vi "tut1_main.vi"() -> ()   [LabVIEW 2014]
uses:
  <vilib>/measure/NI_MABase.lvlib
panel:
  in  "L":dbl(slide)=2e-06 min=1e-06 max=0.001 step=1e-07 scale=1e-06..0.001 scale format="%#.6p"
  out "Current Graph":waveform(dbl)[](graph)
  out "Voltage Graph":waveform(dbl)[](graph)
  out "Control Signal":waveform(dbl)[](graph)
  in  "DutyCycle":dbl(slide)=50.0 caption="Duty Cycle (%)" min=0.0 max=100.0 step=1.0 scale=0.0..100.0 scale format="%#.6p"
  in  "Frequency":dbl(slide)=50.0 caption="Signal Frequency (Hz)" min=0.0 max=5000.0 step=1.0 scale=0.0..100.0 scale format="%#.6p"
  in  "V":dbl(slide)=10.0 caption="Signal Voltage (V)" min=0.0 max=20.0 step=0.1 scale=0.0..20.0 scale format="%#.6p"
  in  "C":dbl(slide)=2e-06 min=1e-06 max=0.001 step=1e-07 scale=1e-06..0.001 scale format="%#.6p"
  in  "R":dbl(slide)=500.0 min=10.0 max=100000.0 step=1.0 scale=10.0..100000.0 scale format="%#.6p"
  in  "stop":bool
  # "PSI3214"
  # "Laboratório de \nInstrumentação Elétrica"
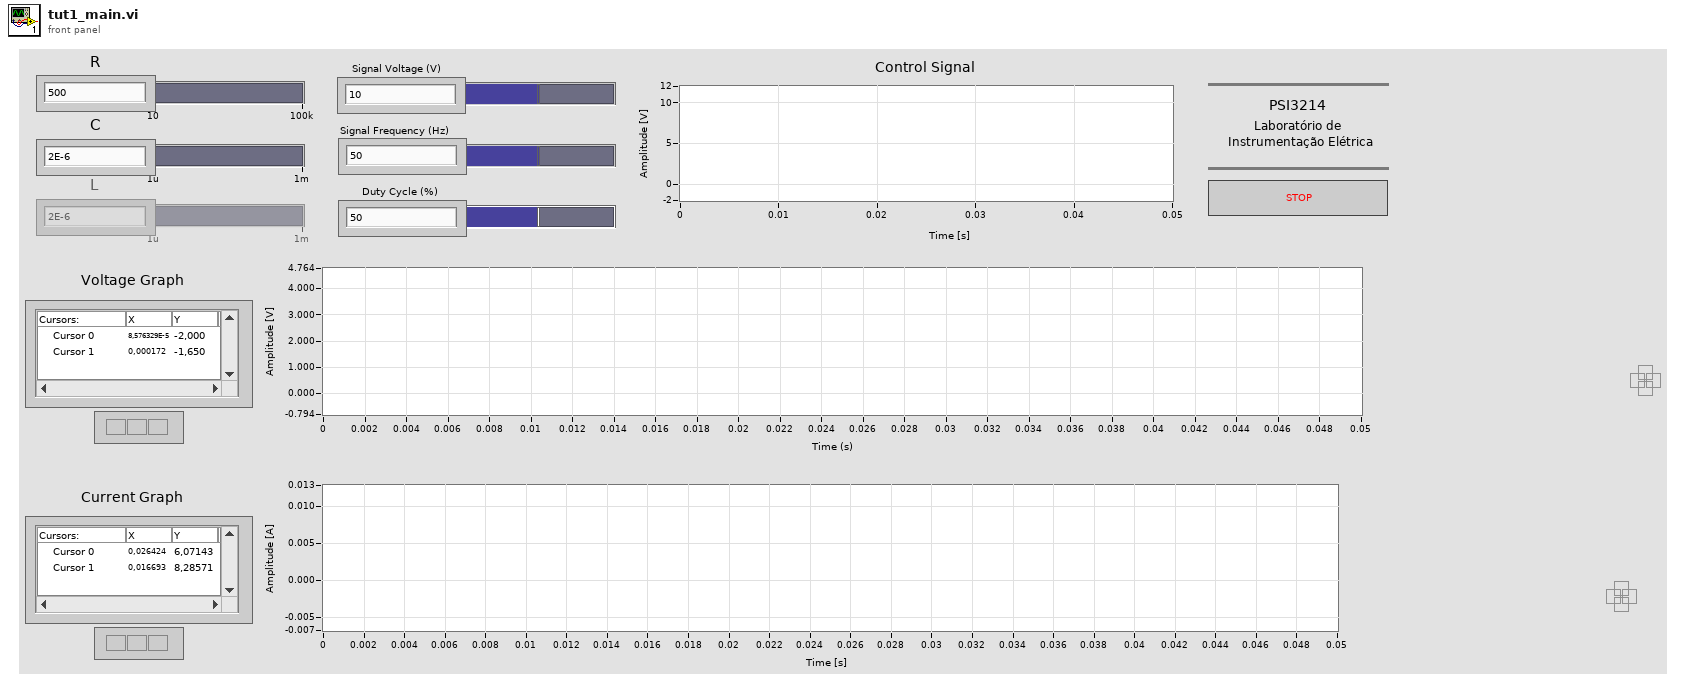
[diagram p1: front panel]
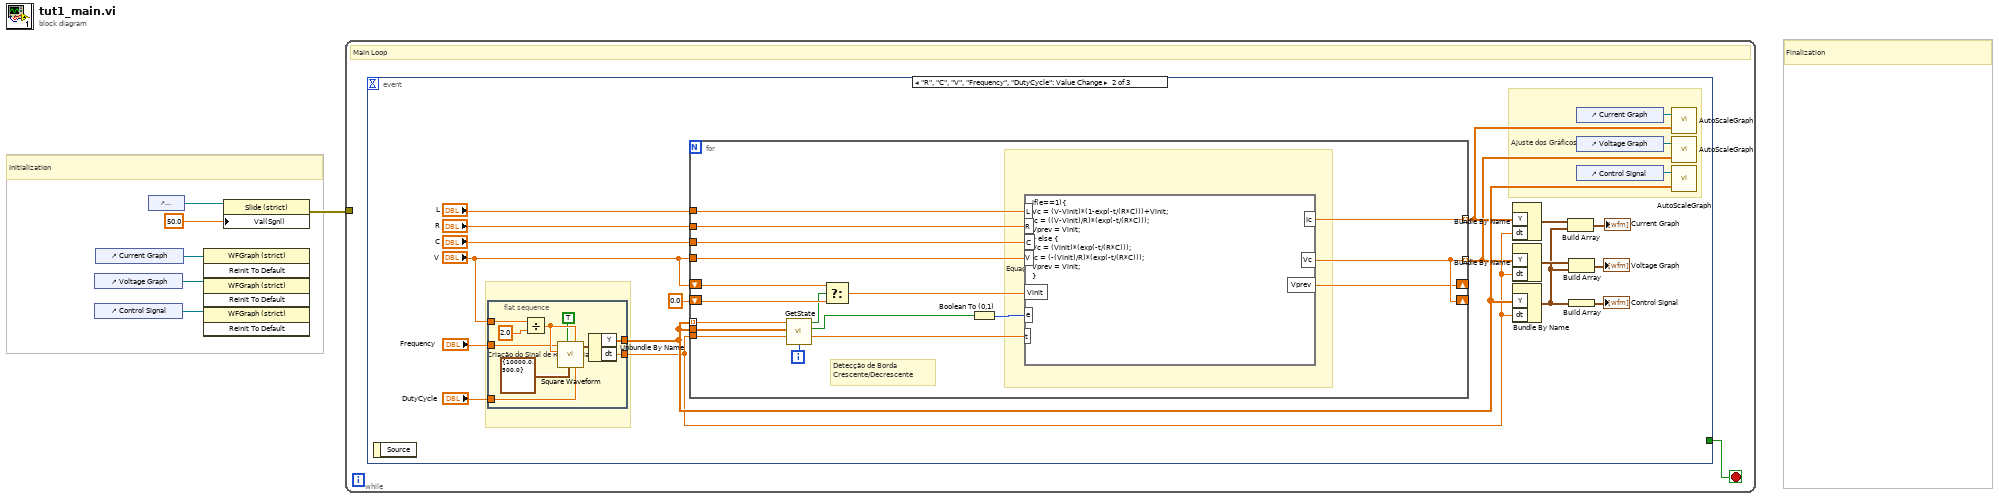
[diagram p0: block diagram]
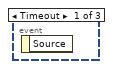
[diagram p2: hidden frame]
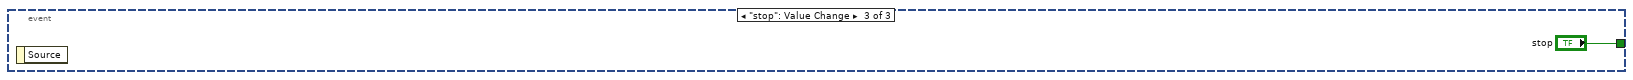
[diagram p3: hidden frame]
diagram:
  # "Finalization"
  # "Initialization"
  n1 = control-ref of="Voltage Graph"() -> (w2:refnum<vi>)
  n2 = control-ref of="Control Signal"() -> (w1:refnum<vi>)
  n3 = control-ref of="Current Graph"() -> (w3:refnum<vi>)
  n4 = control-ref of="Frequency"() -> (w6:refnum<vi>)
  n5 = invoke class="WFGraph (strict)" method="Reinit To Default"(reference=w3) -> ()  [unwired: 2 in, 3 out]
  n6 = invoke class="WFGraph (strict)" method="Reinit To Default"(reference=w2) -> ()  [unwired: 2 in, 3 out]
  n7 = invoke class="WFGraph (strict)" method="Reinit To Default"(reference=w1) -> ()  [unwired: 2 in, 3 out]
  n8 = property class="Slide (strict)"(reference=w6, "Val(Sgnl)"=50.0 ("Value (Signaling)")) -> (error out=w5:errorcluster)  [unwired: 1 in, 1 out]
  n9 = while {
    tunnel: w5 -> [_]
    stop <- w7 stop-if-true
    # "Main Loop"
    n10 = event shown="[1] \"R\", \"C\", \"V\", \"Frequency\", \"DutyCycle\": Value Change" {
      selector: _ -> [_ _ _]
      dyn-events: _ -> [_ _ _]
      timeout: _ -> [_ _ _]
      tunnel: [_ _ "stop"] -> w7
      event Timeout {
        n11 = event-data() -> ()  [unwired: 1 in, 1 out]
      }
      event "R", "C", "V", "Frequency", "DutyCycle": Value Change {
        # "Ajuste dos Gráficos - AutoScale"
        # "Criação do Sinal de Referencia"
        n12 = event-data() -> ()  [unwired: 1 in, 1 out]
        n13 = flat-sequence {
          tunnel: "V" -> [w33]
          tunnel: "Frequency" -> [w32]
          tunnel: "DutyCycle" -> [w31]
          tunnel: [w30] -> w16
          tunnel: [w29] -> w14
          frame #0 {
            n14 = Divide(x=w33, y=2.0) -> (x/y=w35:dbl)
            n15 = call <vilib>:"Square Waveform.vi"("duty cycle (%)"=w31, "offset"=w35, "sampling info"=cluster{"Fs":dbl, "#s":dbl} {"Fs"=10000.0, "#s"=500.0}, "reset signal"=TRUE, "amplitude"=w35, "frequency"=w32) -> ("signal out"=w34:waveform(dbl))  [unwired: 4 in, 1 out]
            n16 = Unbundle By Name(w34) -> ("Y"=w30:dbl[], "dt"=w29:dbl)
          }
        }
        n17 = for {
          tunnel: "R" -> [w55]
          tunnel: "C" -> [w54]
          tunnel: "V" -> [w50]
          tunnel: [w51] -> w9 mode=indexing
          tunnel: w16 -> [w52] mode=indexing
          tunnel: w16 -> [w53]
          shift-right: [w51] -> _
          shift-left: 0.0 ("y") -> [w46]
          shift-right: [w42] -> _
          shift-left: "V" -> [w45]
          tunnel: w14 -> [w48]
          tunnel: "L" -> [w41]
          tunnel: [w40] -> w10 mode=indexing
          i -> [w49]
          # "Detecção de Borda\nCrescente/Decrescente"
          # "Equações de Carga e Descarga - Circuitos de Primeira Ordem"
          n18 = call "GetState.vi"("Array Element"=w52, "Array"=w53, "dt"=w48, "Loop Iteration"=w49) -> ("Change State"=w44:bool, "Rising/Falling Edge"=w39:bool, "t"=w47:dbl)  [unwired: 3 in]
          n19 = Select(t=w45, s=w44, f=w46) -> (s? t:f=w43:dbl)
          n20 = Boolean To (0,1)(Boolean=w39) -> (0, 1=w38:i16)
          n21 = formula code="if(e==1){\nVc = (V-Vinit)*(1-exp(-t/(R*C)))+Vinit;\nIc = ((V-Vinit)/R)*(exp(-t/(R*C)));\nVprev = Vinit;\n} else {\nVc = (Vinit)*(exp(-t/(R*C)));\nIc = (-(Vinit)/R)*(exp(-t/(R*C)));\nVprev = Vinit;\n}"("R"=w55, "C"=w54, "V"=w50, "t"=w47, "Vinit"=w43, "L"=w41, "e"=w38) -> ("Vc"=w51:dbl, "Vprev"=w42:dbl, "Ic"=w40:dbl)
        }
        n22 = Bundle By Name("Y"=w10, "dt"=w14) -> (w23:waveform(dbl))  [unwired: 1 in]
        n23 = Bundle By Name("Y"=w9, "dt"=w14) -> (w22:waveform(dbl))  [unwired: 1 in]
        n24 = Bundle By Name("Y"=w16, "dt"=w14) -> (w20:waveform(dbl))  [unwired: 1 in]
        n25 = Build Array(w23, w20) -> (→"Current Graph":waveform(dbl)[])
        n26 = Build Array(w22, w20) -> (→"Voltage Graph":waveform(dbl)[])
        n27 = Build Array(w20) -> (→"Control Signal":waveform(dbl)[])
        n28 = control-ref of="Current Graph"() -> (w13:refnum<vi>)
        n29 = control-ref of="Voltage Graph"() -> (w12:refnum<vi>)
        n30 = control-ref of="Control Signal"() -> (w11:refnum<vi>)
        n31 = call "AutoScaleGraph.vi"("Array"=w10, "WaveformGraph in"=w13) -> ()  [unwired: 1 in]
        n32 = call "AutoScaleGraph.vi"("Array"=w9, "WaveformGraph in"=w12) -> ()  [unwired: 1 in]
        n33 = call "AutoScaleGraph.vi"("Array"=w16, "WaveformGraph in"=w11) -> ()  [unwired: 1 in]
      }
      event "stop": Value Change {
        n34 = event-data() -> ()  [unwired: 1 in, 1 out]
      }
    }
  }
